vi "ovenCtrl_Na.vi"(6 "Error In (no error)":errorcluster, 9 "Temperature Log Interval (s)":dbl=20.0, 10 "Port Number Heater 1":u16=2000, 11 "IP Address Heater 1":string="192.168.12.200") -> (0 "Error Out":errorcluster, 3 "T1 (C)":dbl=214.9 format="%.2f")   [LabVIEW 2013, in "NaOvenControlV6SubVIs.lvlib"]
uses:
  VIs/NaOvenControlV6SubVIs.lvlib
panel:
  out "Oven Ramp Down Status (ON/OFF)":bool
  in  "Process":u16(ring)=1 items=["Log Temperature", "Wait - ON - Log", "OFF - Log", "OFF - Wait -ON - Log"]
  in  "Next Weekday":bool
  in  "Year":i32=2021 min=2019 step=1
  in  "Month":i32=3 min=1 max=12 step=1
  in  "Day":i32=23 min=1 max=31 step=1
  out "Oven Ramp Up Status (ON/OFF)":bool
  out "Oven Ramp ON Time":string="7:15 AM"
  out "Oven Ramp ON Date":string="Monday, March 22, 2021"
  in  "Turn ON Minute":i32=15 min=0 max=59 step=1
  in  "Turn ON Hour":i32=7 min=0 max=23 step=1
  in  "Final Hot Heater 1 Temperature (C)":dbl=215.0 min=20.0 max=260.0 step=0.1
  in  "Ramp Up Duration (min)":dbl=120.0
  in  "Set To Room Temp?":bool
  in  "Additional Temp for Heater 2":dbl=45.0
  in  "Ramp Down Duration (min)":dbl=100.0
  in  "Final Cold Heater 1 Temperature (C)":dbl=10.0 min=5.0 max=260.0 step=0.1 format="%.2f"
  out "Update to Influx (T2)":bool
  out "Update to Influx (T1)":bool
  out "T2 (C)":dbl=260.0 format="%.2f"
  in  "Port Number Heater 2":u16=2000
  in  "IP Address Heater 2":string="192.168.12.201"
  # "Common Inputs"
  # "Outputs"
  # "The Temperature and Influx update status is disabled during Ramp Up and Down"
  # "Turn ON Inputs"
  # "Ramp ON time is not visible when not scheduled"
  # "Tun OFF Inputs"
  # "Diagnosis"
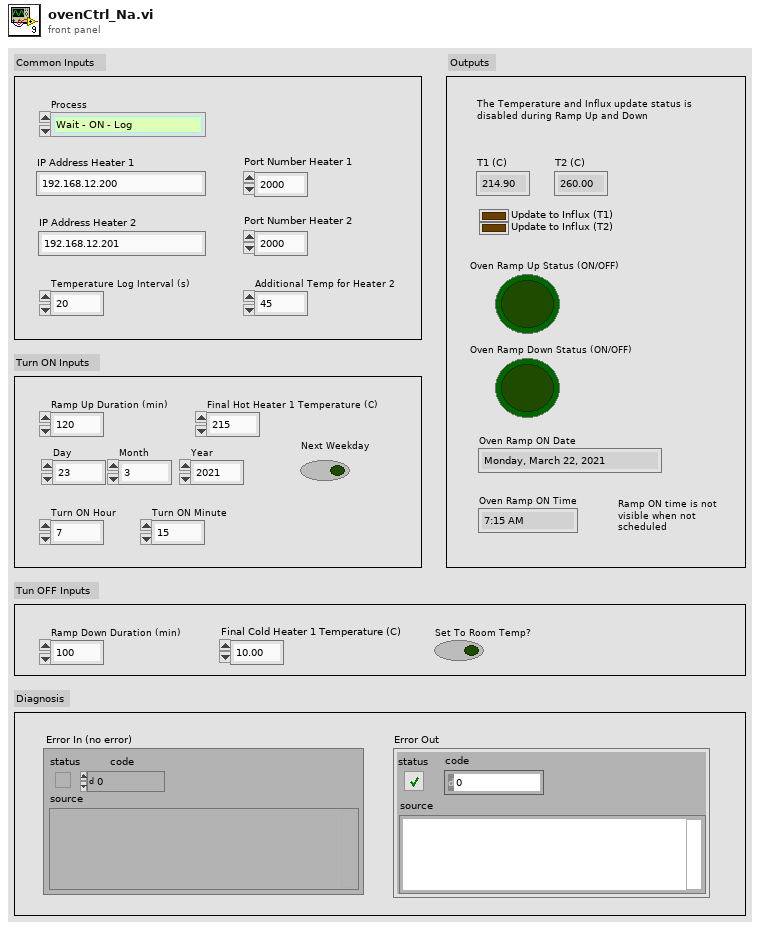
[diagram p1: front panel]
types:
  T1 = typedef "LVDateTimeRec.ctl" = cluster{"fractional second":dbl, "second":i32, "minute":i32, "hour":i32, "day of month":i32, "month":i32, "year":i32, "day of week":i32, "day of year":i32, "DST":i32}
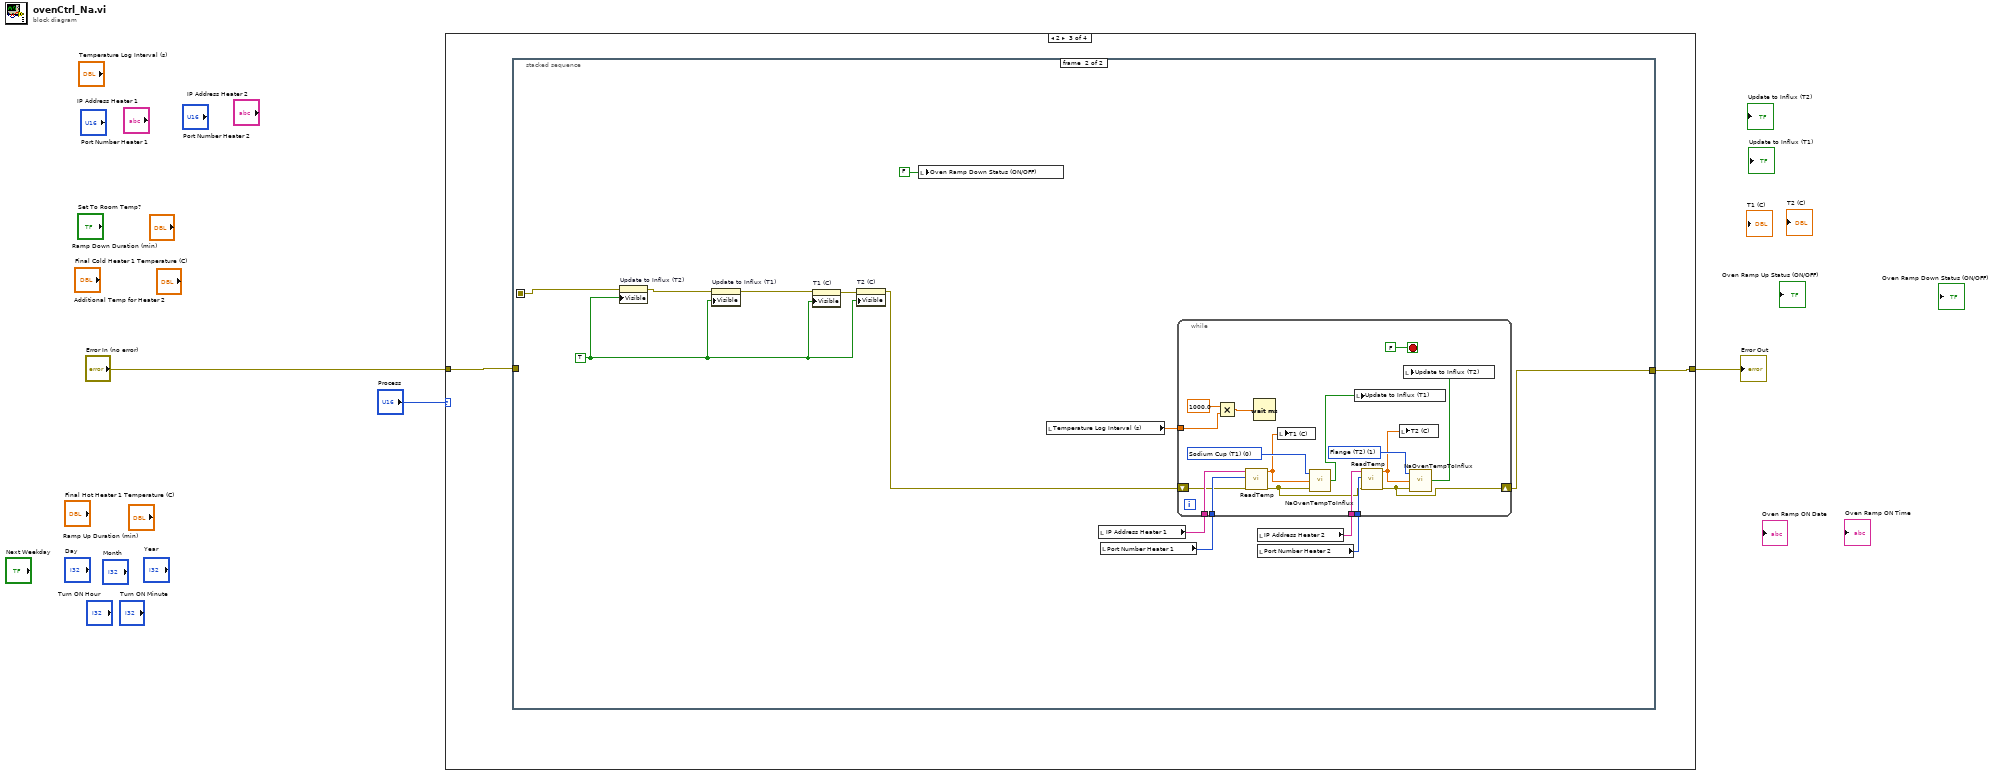
[diagram p0: block diagram]
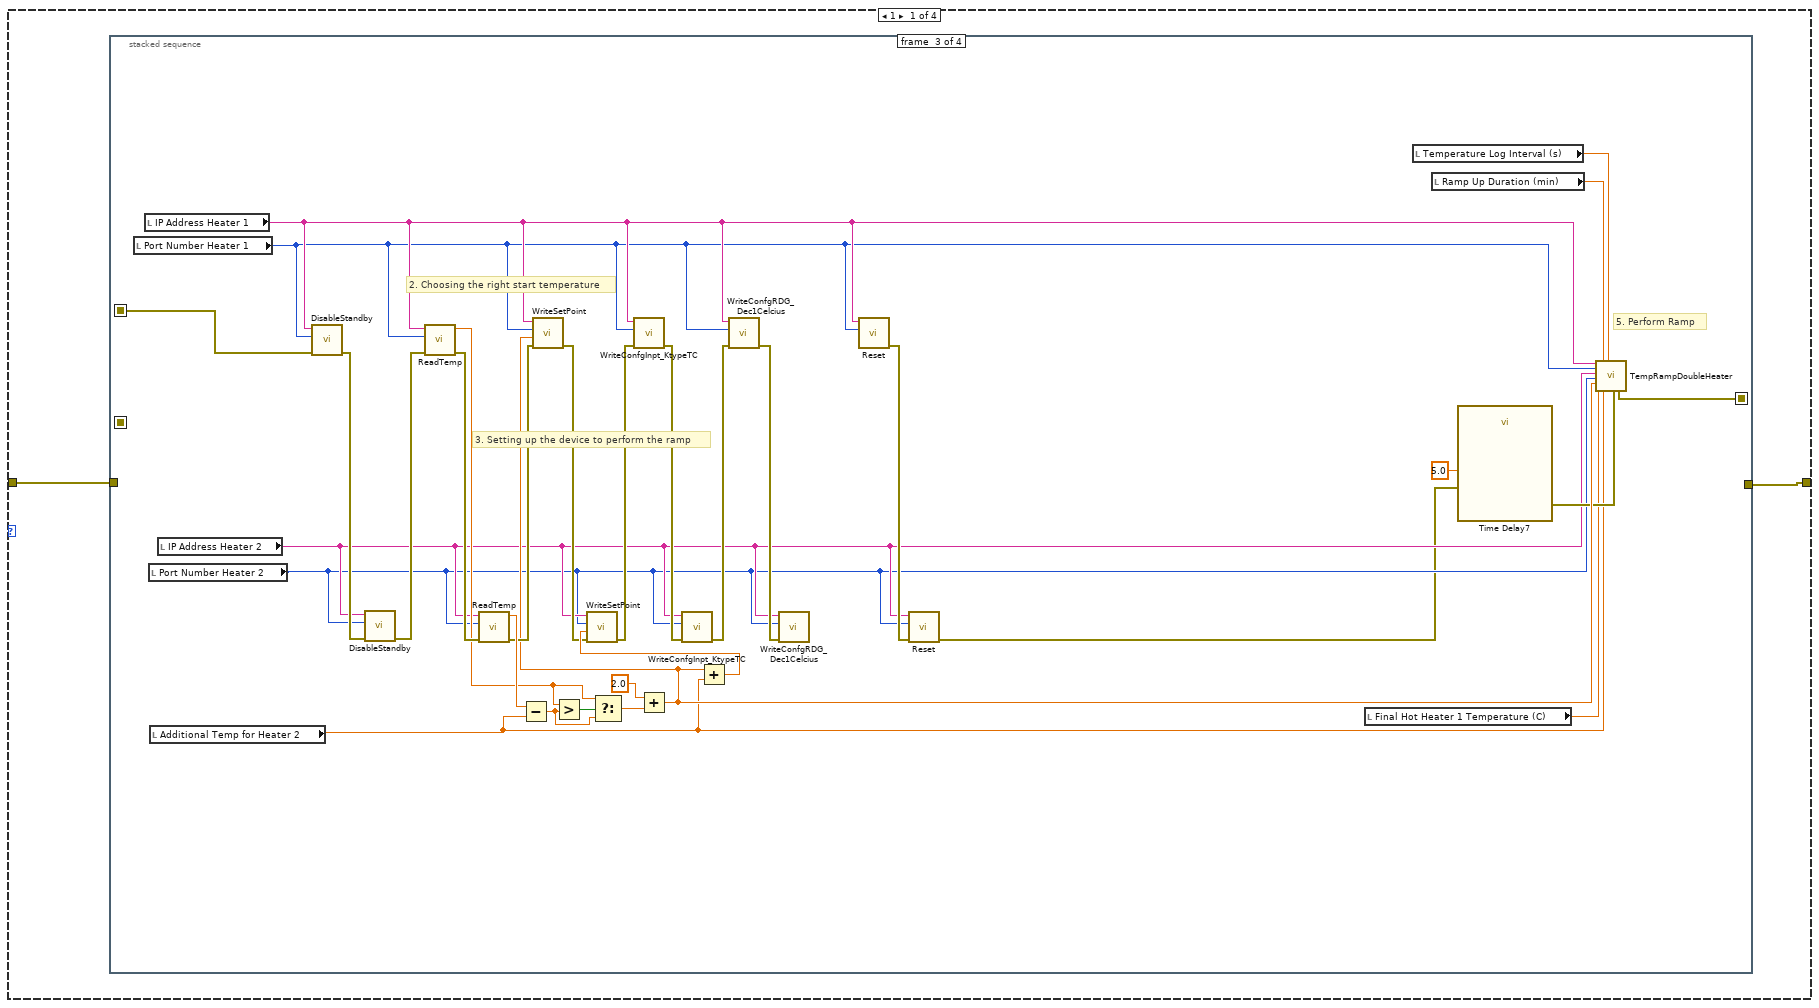
[diagram p2: hidden frame]
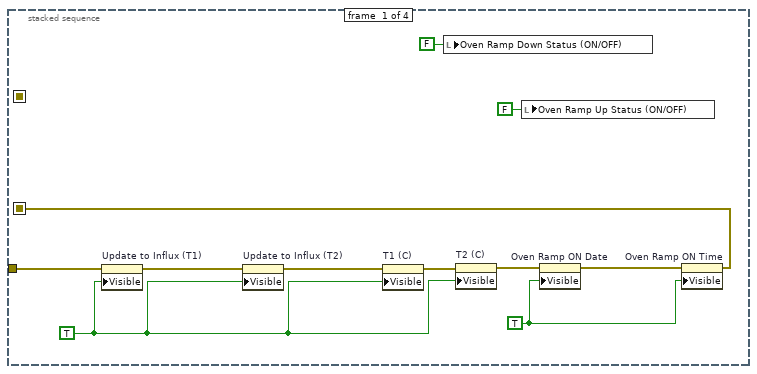
[diagram p3: hidden frame]
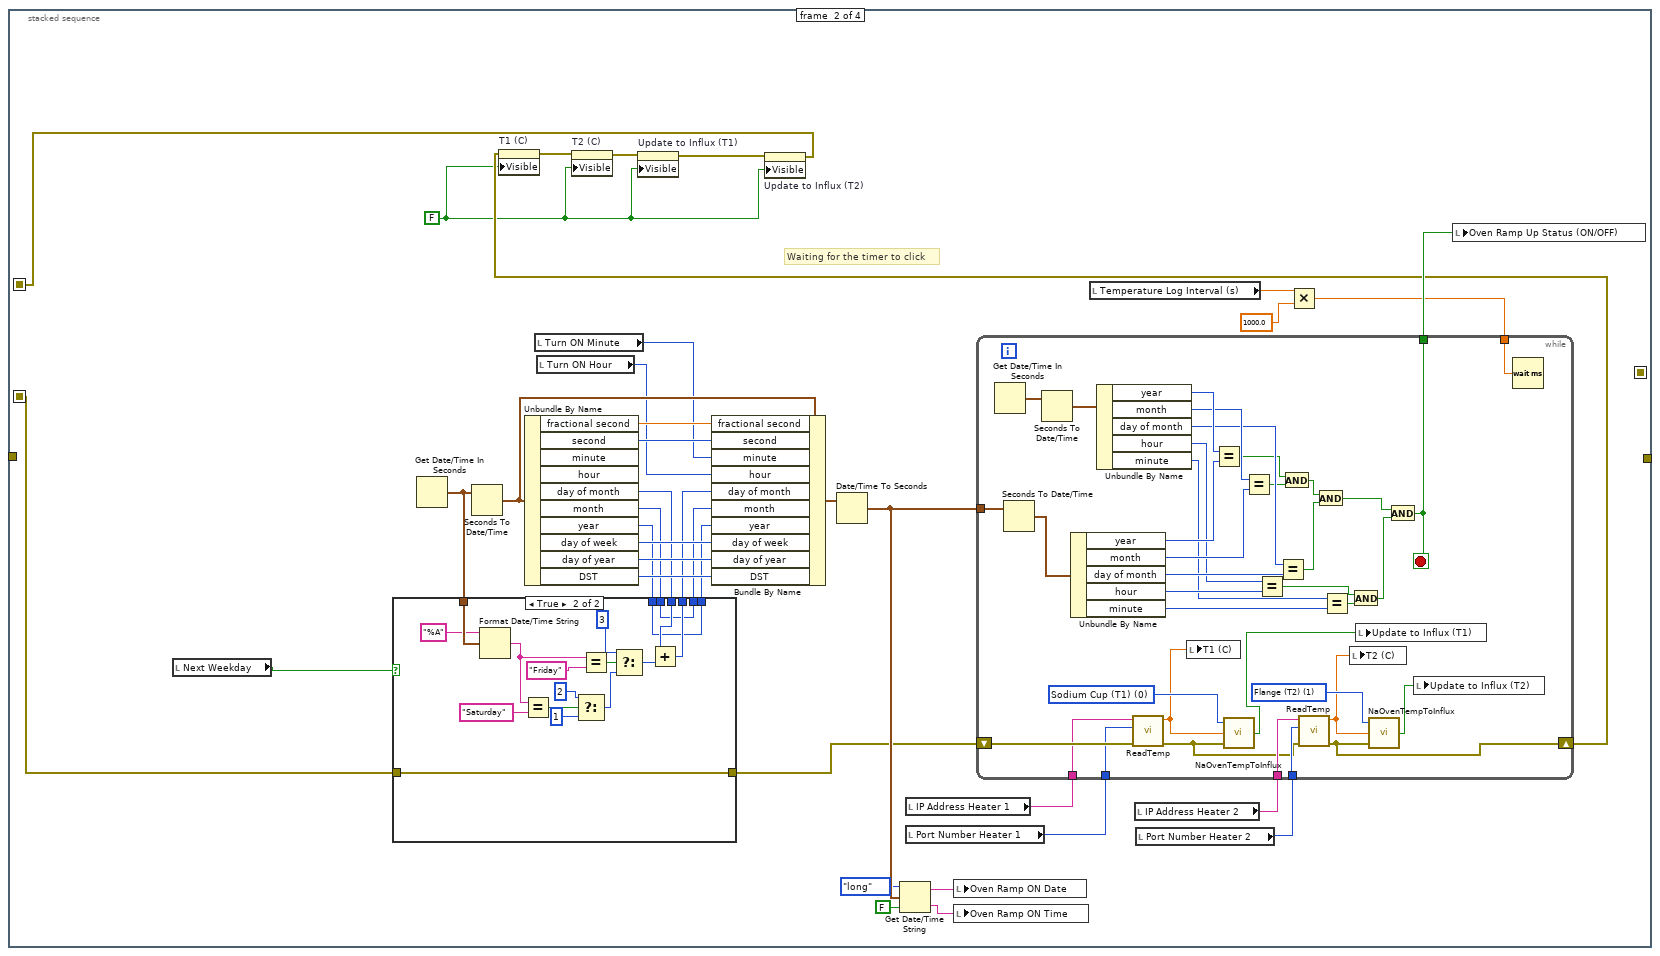
[diagram p4: hidden frame]
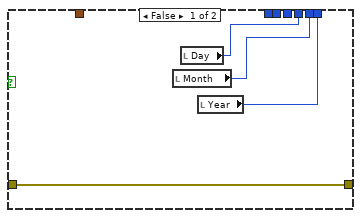
[diagram p5: hidden frame]
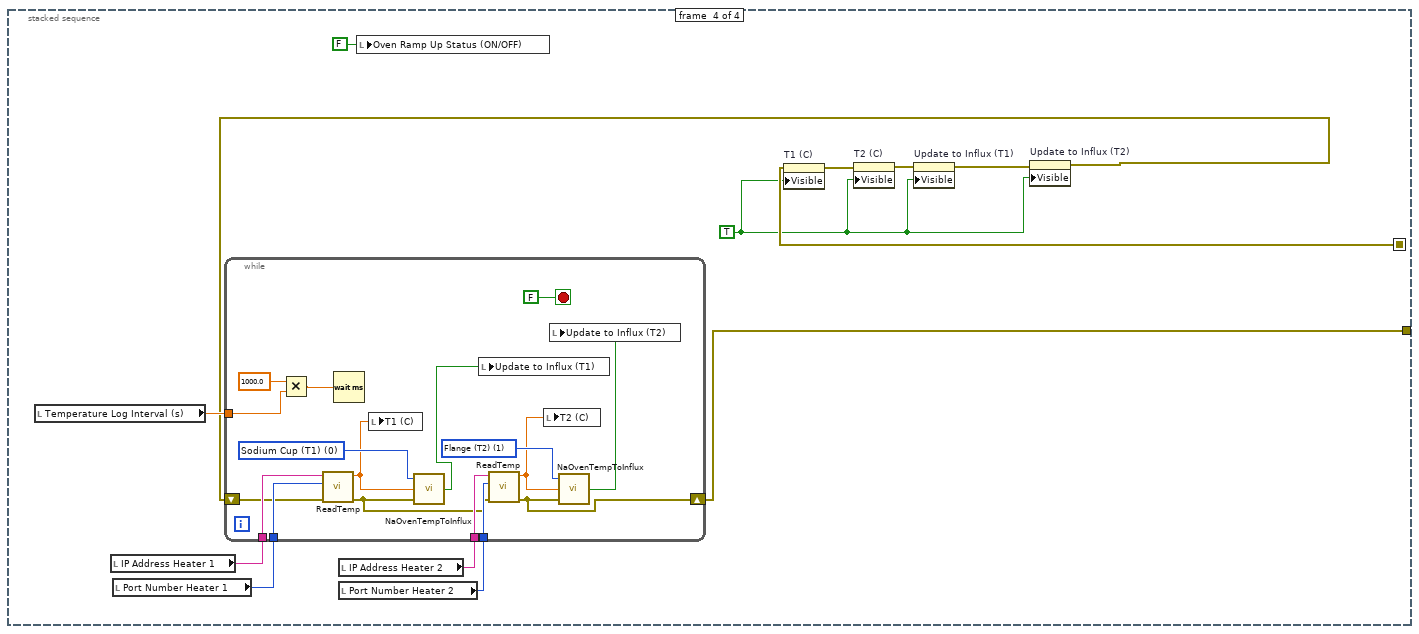
[diagram p6: hidden frame]
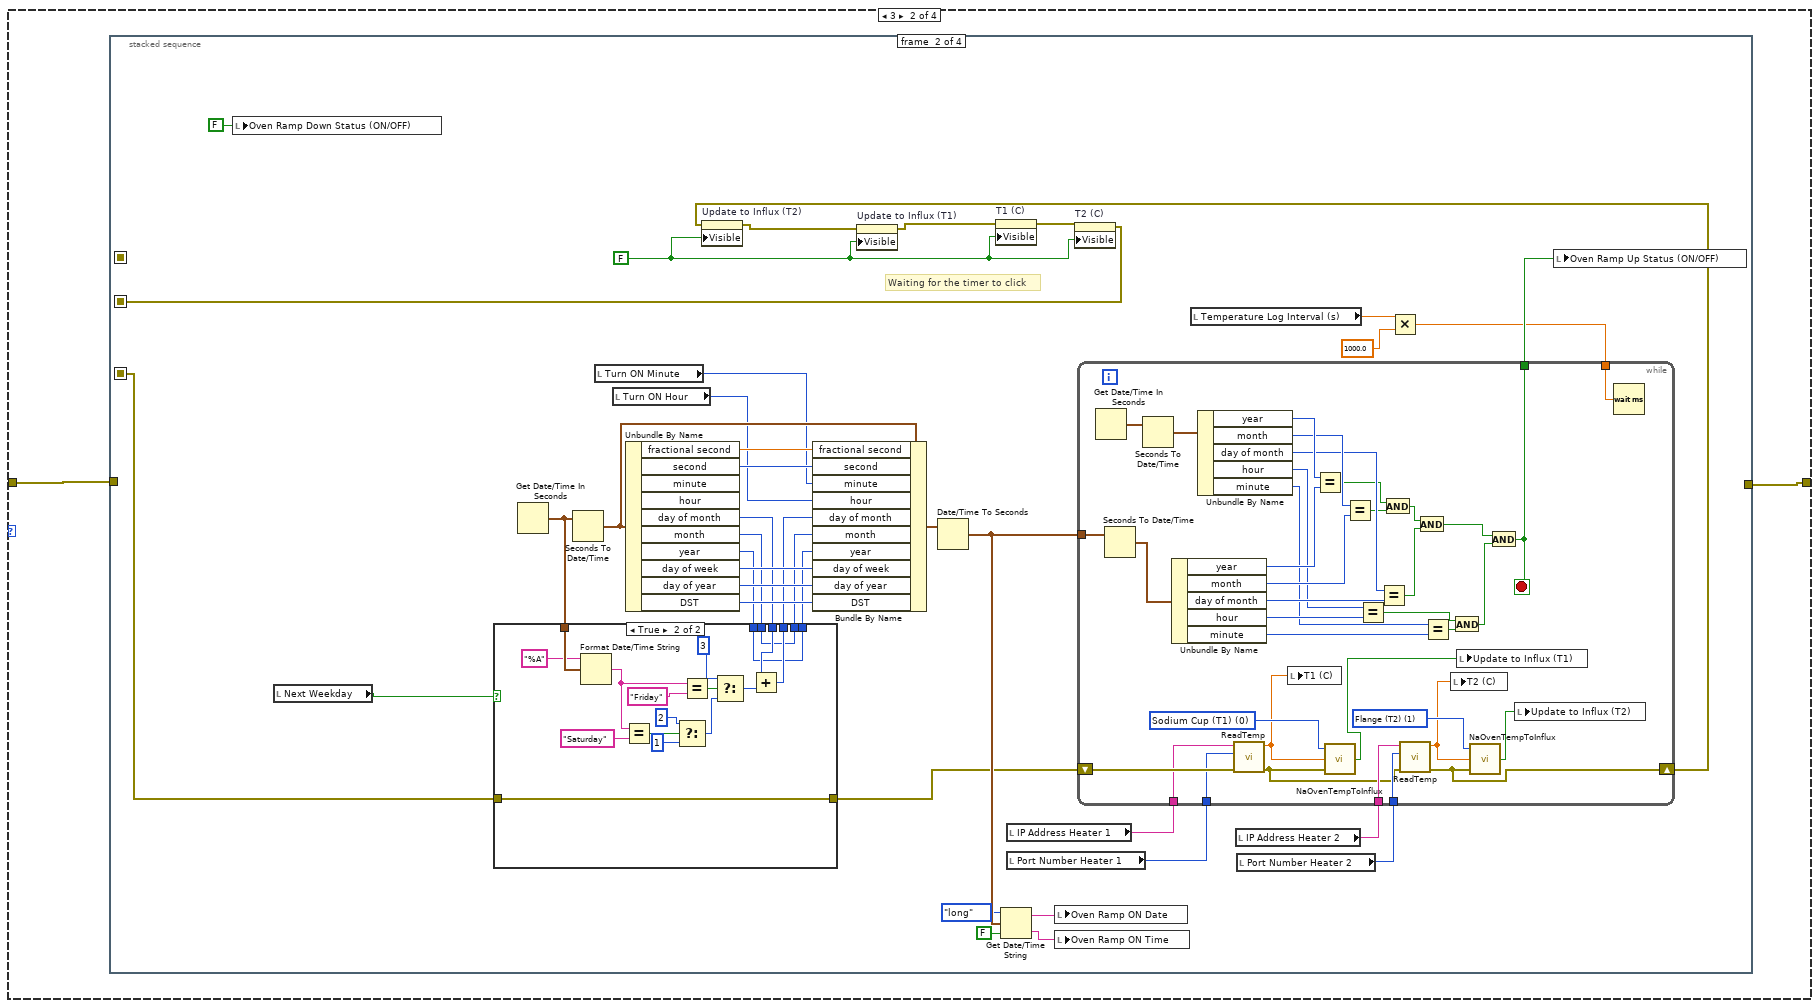
[diagram p7: hidden frame]
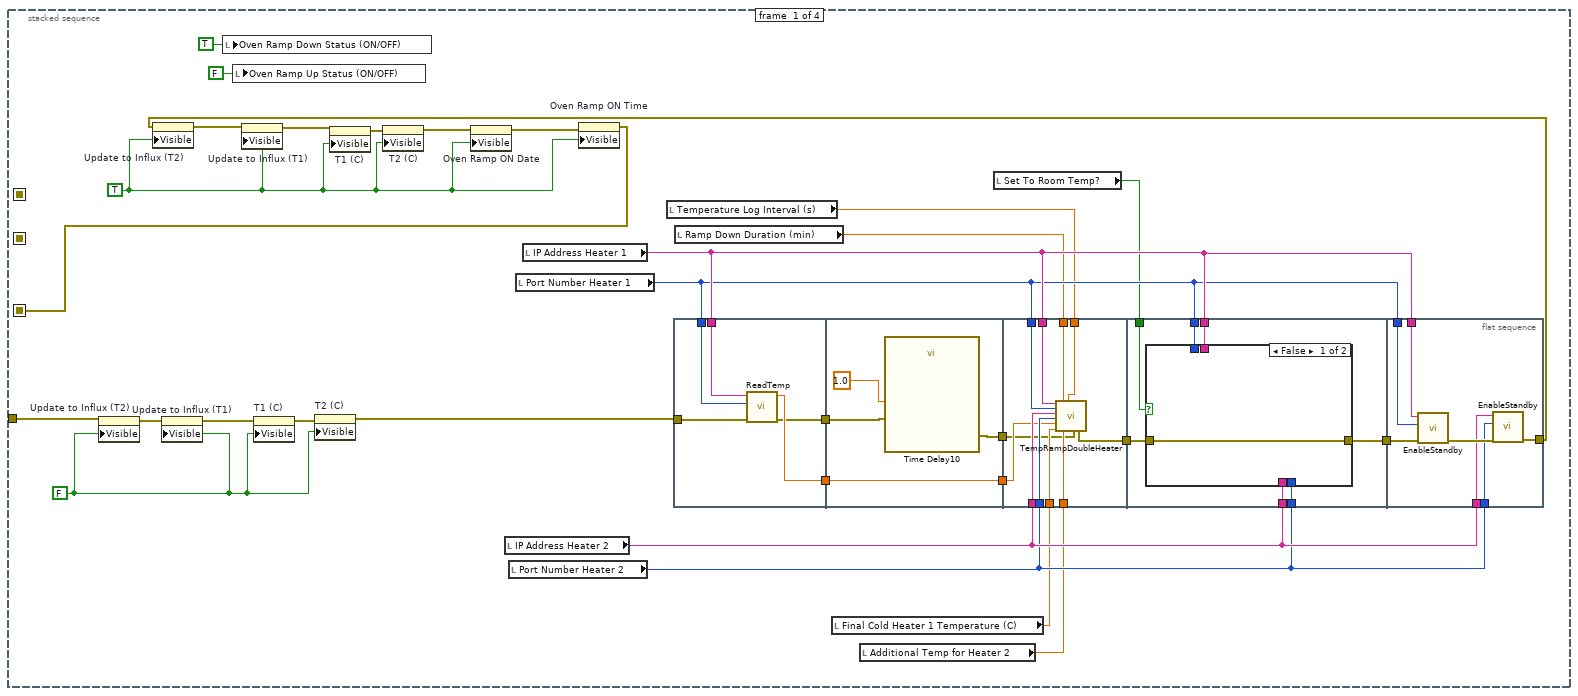
[diagram p8: hidden frame]
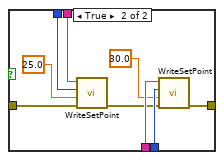
[diagram p9: hidden frame]
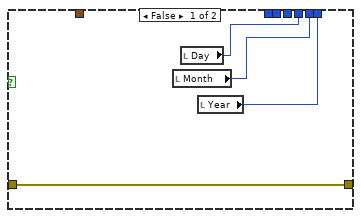
[diagram p10: hidden frame]
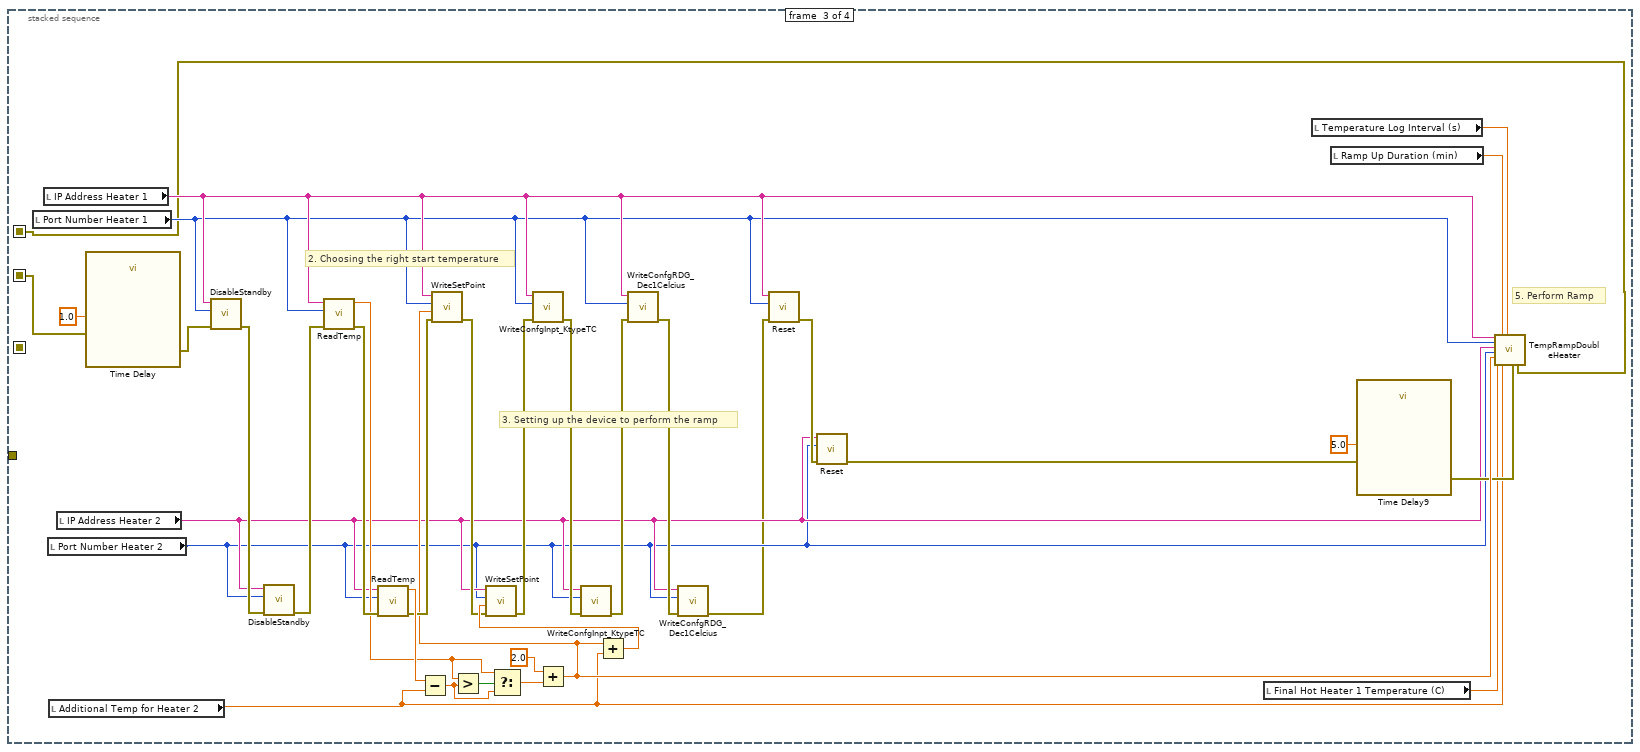
[diagram p11: hidden frame]
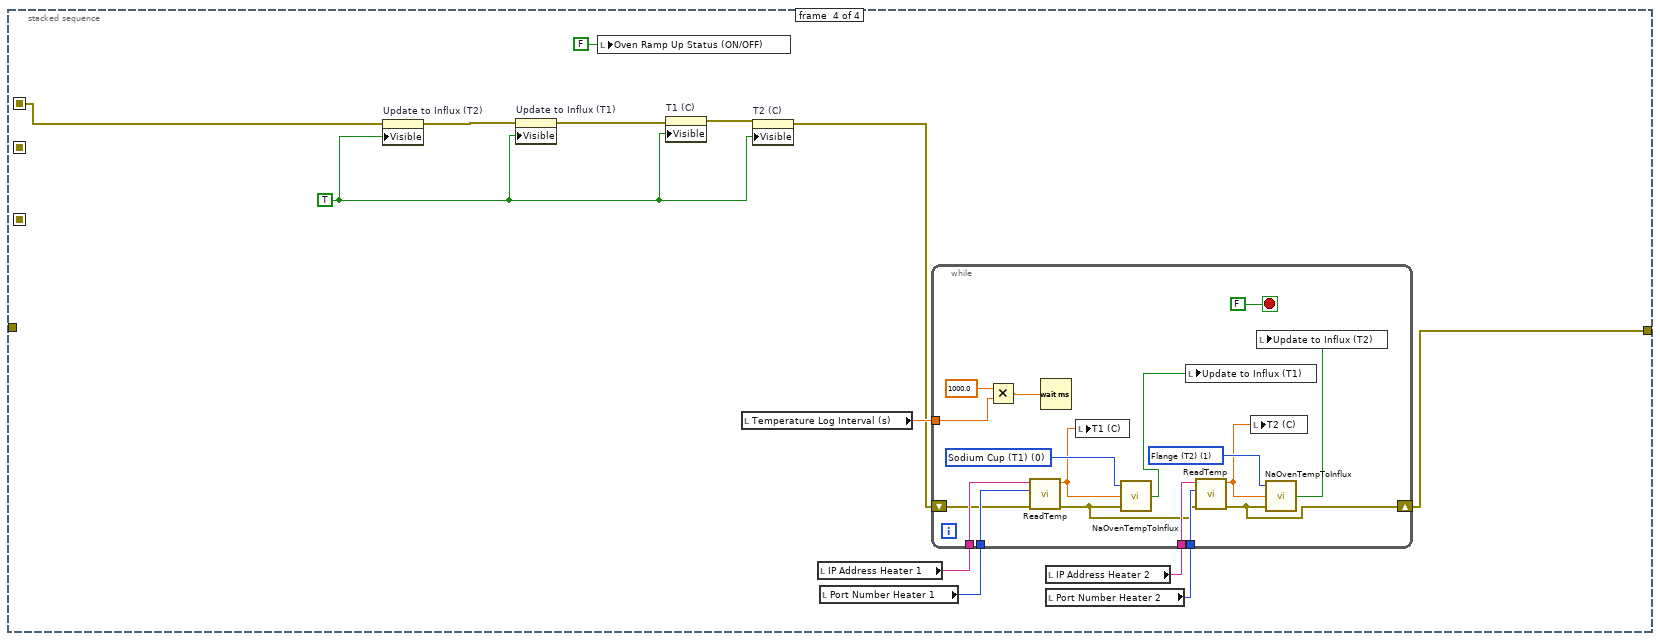
[diagram p12: hidden frame]
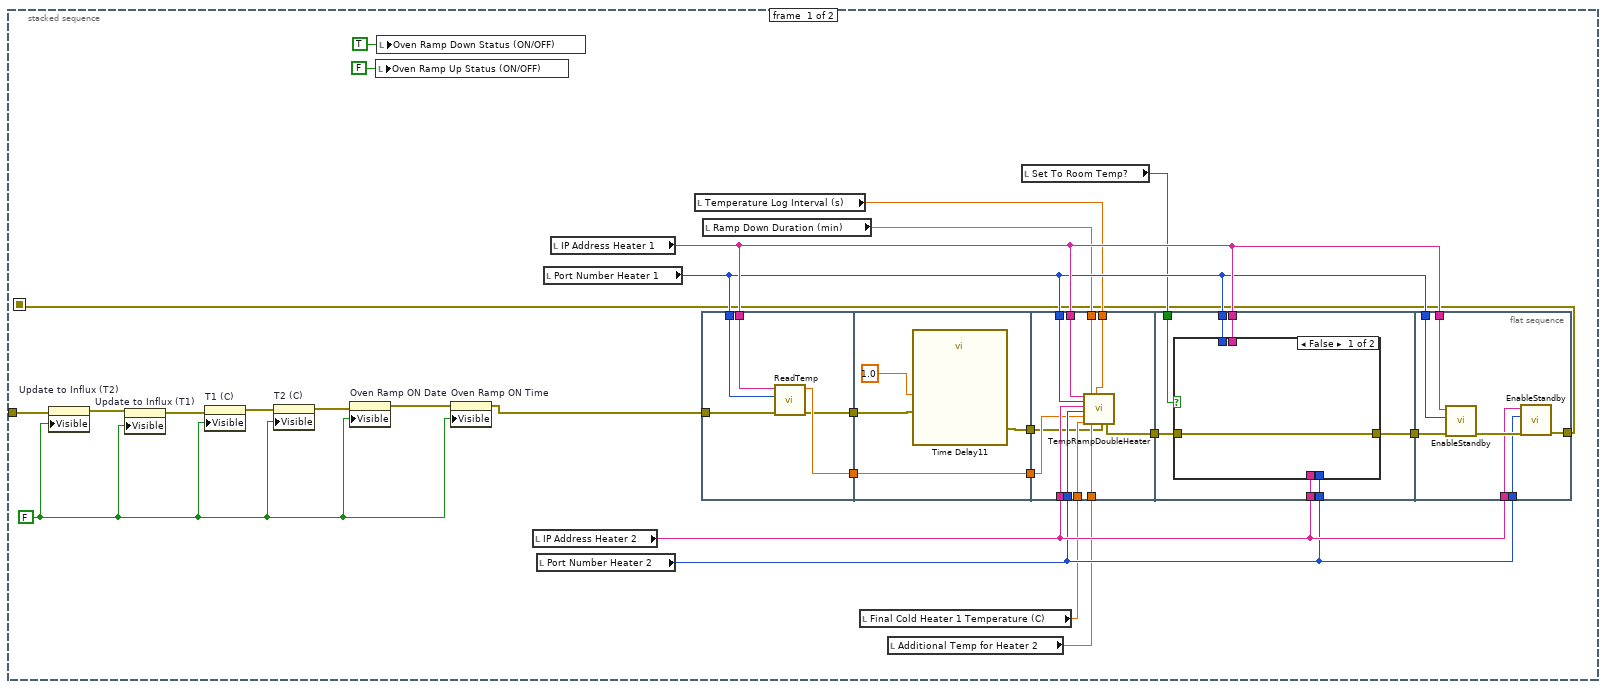
[diagram p13: hidden frame]
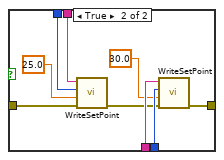
[diagram p14: hidden frame]
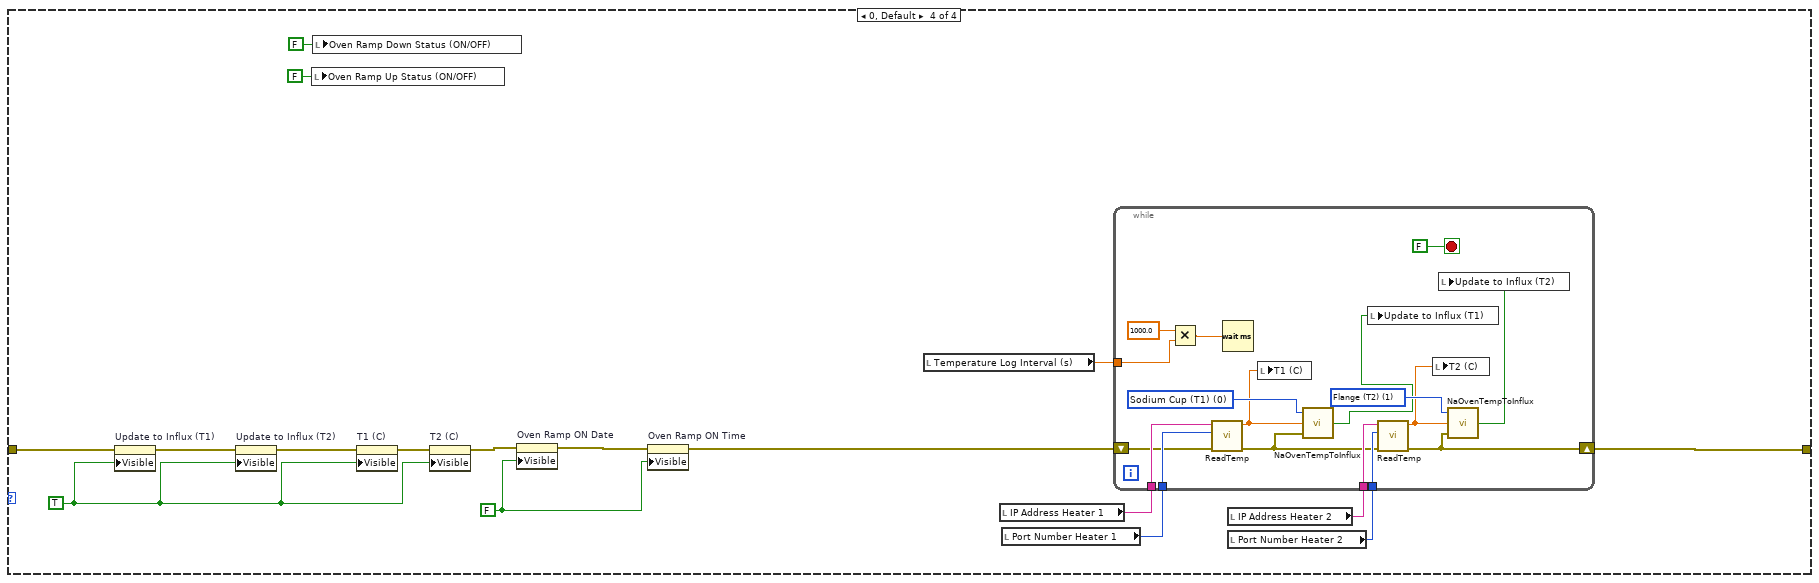
[diagram p15: hidden frame]
diagram:
  n1 = case shown="2" "Process" {
    tunnel: [w4 w174 w412 w530] -> w3
    tunnel: "Error In (no error)" -> [w5 w175 w413 w522]
    frame 1 {
      n2 = stacked-sequence {
        seq-local: [_ w18 _ _] -> [_ _ w115 _]
        seq-local: [_ _ w114 _] -> [_ _ _ w149]
        seq-local: [w7 _ _ _] -> [_ w25 _ _]
        tunnel: w5 -> [w14 _ _ _]
        tunnel: [_ _ _ w151] -> w4
        frame #0 {
          w6 = TRUE ("Visible")
          w10 = TRUE ("Visible")
          n3 = property on="Update to Influx (T1)" class="Bool (strict)"(error in=w14, "Visible"=w10) -> (error out=w13:errorcluster)  [unwired: 1 in, 1 out]
          n4 = property on="Update to Influx (T2)" class="Bool (strict)"(error in=w13, "Visible"=w10) -> (error out=w12:errorcluster)  [unwired: 1 in, 1 out]
          n5 = property on="T1 (C)" class="DigNum (strict)"(error in=w12, "Visible"=w10) -> (error out=w11:errorcluster)  [unwired: 1 in, 1 out]
          n6 = local write "Oven Ramp Down Status (ON/OFF)"(FALSE ("Oven Ramp Down Status (ON/OFF)")) -> ()
          n7 = property on="T2 (C)" class="DigNum (strict)"(error in=w11, "Visible"=w10) -> (error out=w9:errorcluster)  [unwired: 1 in, 1 out]
          n8 = local write "Oven Ramp Up Status (ON/OFF)"(FALSE ("Oven Ramp Up Status (ON/OFF)")) -> ()
          n9 = property on="Oven Ramp ON Date" class="Str"(error in=w9, "Visible"=w6) -> (error out=w8:errorcluster)  [unwired: 1 in, 1 out]
          n10 = property on="Oven Ramp ON Time" class="Str"(error in=w8, "Visible"=w6) -> (error out=w7:errorcluster)  [unwired: 1 in, 1 out]
        }
        frame #1 {
          w17 = FALSE ("Visible")
          # "Waiting for the timer to click"
          n11 = local read "Next Weekday"() -> (w35:bool)
          n12 = Get Date/Time In Seconds() -> (seconds since 1Jan1904=w47:timestamp)
          n13 = Seconds To Date/Time(time stamp (now)=w47) -> (date time rec=w49:T1)  [unwired: 1 in]
          n14 = Unbundle By Name(w49) -> ("fractional second"=w54:dbl, "second"=w53:i32, "day of month"=w46:i32, "month"=w44:i32, "year"=w42:i32, "day of week"=w52:i32, "day of year"=w51:i32, "DST"=w50:i32)  [unwired: 2 out]
          n15 = case shown="True" w35 {
            tunnel: w47 -> [_ w75]
            tunnel: w46 -> [_ w64]
            tunnel: [w57 w62] -> w45
            tunnel: w44 -> [_ w61]
            tunnel: [w56 w61] -> w43
            tunnel: w42 -> [_ w60]
            tunnel: [w55 w60] -> w41
            tunnel: w25 -> [w58 w59]
            tunnel: [w58 w59] -> w36
            frame False {
              n16 = local read "Month"() -> (w56:i32)
              n17 = local read "Day"() -> (w57:i32)
              n18 = local read "Year"() -> (w55:i32)
            }
            frame True {
              n19 = Format Date/Time String(time format string (%c)="%A", seconds (now)=w75) -> (date/time string=w72:string)  [unwired: 1 in]
              n20 = Equal?(x=w72, y="Saturday") -> (x = y?=w68:bool)
              n21 = Select(t=2, s=w68, f=1) -> (s? t:f=w65:i32)
              n22 = Equal?(x=w72, y="Friday") -> (x = y?=w70:bool)
              n23 = Select(t=3, s=w70, f=w65) -> (s? t:f=w63:i32)
              n24 = Add(x=w64, y=w63) -> (x+y=w62:i32)
            }
          }
          n25 = local read "Turn ON Minute"() -> (w24:i32)
          n26 = local read "Turn ON Hour"() -> (w23:i32)
          n27 = Bundle By Name(cluster=w49, "fractional second"=w54, "second"=w53, "minute"=w24, "hour"=w23, "day of month"=w45, "month"=w43, "year"=w41, "day of week"=w52, "day of year"=w51, "DST"=w50) -> (w48:T1)
          n28 = Date/Time To Seconds(2:w48) -> (0:w39:timestamp)  [unwired: 1 in]
          n29 = Get Date/Time String(date format (0)=enum16{"short", "long", "abbreviated"}."long", seconds (now)=w39, want seconds? (F)=FALSE) -> (date string=w34:string, time string=w33:string)
          n30 = local read "IP Address Heater 1"() -> (w29:string)
          n31 = local read "Port Number Heater 1"() -> (w28:u16)
          n32 = local write "Oven Ramp ON Date"(w34) -> ()
          n33 = local write "Oven Ramp ON Time"(w33) -> ()
          n34 = local read "Temperature Log Interval (s)"() -> (w31:dbl)
          n35 = local read "IP Address Heater 2"() -> (w26:string)
          n36 = local read "Port Number Heater 2"() -> (w27:u16)
          n37 = Multiply(x=w31, y=1000.0) -> (x*y=w30:dbl)
          n38 = while {
            tunnel: w39 -> [w111]
            tunnel: [w90] -> w40
            shift-right: [w76] -> w22
            shift-left: w36 -> [w86]
            tunnel: w30 -> [w89]
            tunnel: w29 -> [w83]
            tunnel: w28 -> [w82]
            tunnel: w27 -> [w81]
            tunnel: w26 -> [w80]
            stop <- w90 stop-if-true
            w87 = u16 1 items=["Sodium Cup (T1)", "Flange (T2)"] ("Thermocouple")
            w88 = u16 0 items=["Sodium Cup (T1)", "Flange (T2)"] ("Thermocouple")
            n39 = Get Date/Time In Seconds() -> (seconds since 1Jan1904=w112:timestamp)
            n40 = Seconds To Date/Time(time stamp (now)=w111) -> (date time rec=w110:T1)  [unwired: 1 in]
            n41 = Seconds To Date/Time(time stamp (now)=w112) -> (date time rec=w109:T1)  [unwired: 1 in]
            n42 = Unbundle By Name(w110) -> ("year"=w107:i32, "month"=w105:i32, "day of month"=w103:i32, "hour"=w101:i32, "minute"=w99:i32)
            n43 = Unbundle By Name(w109) -> ("year"=w108:i32, "month"=w106:i32, "day of month"=w104:i32, "hour"=w102:i32, "minute"=w100:i32)
            n44 = call "ReadTemp.vi"("error in (no error)"=w86, "Port Number"=w82, "IP Address"=w83) -> ("error out"=w77:errorcluster, "Temperature"=w85:dbl)  [unwired: 7 in]
            n45 = local write "T1 (C)"(w85) -> ()
            n46 = Equal?(x=w108, y=w107) -> (x = y?=w98:bool)
            n47 = call "NaOvenTempToInflux.vi"("error in (no error)"=w77, "Temperature Input"=w85, "Thermocouple"=w88) -> ("InfluxDB Comm Error"=w79:bool)  [unwired: 1 in, 1 out]
            n48 = Equal?(x=w106, y=w105) -> (x = y?=w97:bool)
            n49 = Equal?(x=w102, y=w101) -> (x = y?=w96:bool)
            n50 = Equal?(x=w104, y=w103) -> (x = y?=w93:bool)
            n51 = And(x=w98, y=w97) -> (x .and. y?=w94:bool)
            n52 = call "ReadTemp.vi"("error in (no error)"=w77, "Port Number"=w81, "IP Address"=w80) -> ("error out"=w76:errorcluster, "Temperature"=w84:dbl)  [unwired: 7 in]
            n53 = And(x=w94, y=w93) -> (x .and. y?=w92:bool)
            n54 = Equal?(x=w100, y=w99) -> (x = y?=w95:bool)
            n55 = local write "T2 (C)"(w84) -> ()
            n56 = And(x=w96, y=w95) -> (x .and. y?=w91:bool)
            n57 = local write "Update to Influx (T1)"(w79) -> ()
            n58 = call "NaOvenTempToInflux.vi"("error in (no error)"=w76, "Temperature Input"=w84, "Thermocouple"=w87) -> ("InfluxDB Comm Error"=w78:bool)  [unwired: 1 in, 1 out]
            n59 = And(x=w92, y=w91) -> (x .and. y?=w90:bool)
            n60 = local write "Update to Influx (T2)"(w78) -> ()
            n61 = Wait (ms)(milliseconds to wait=w89) -> ()  [unwired: 1 out]
          }
          n62 = property on="T1 (C)" class="DigNum (strict)"(error in=w22, "Visible"=w17) -> (error out=w21:errorcluster)  [unwired: 1 in, 1 out]
          n63 = property on="T2 (C)" class="DigNum (strict)"(error in=w21, "Visible"=w17) -> (error out=w20:errorcluster)  [unwired: 1 in, 1 out]
          n64 = property on="Update to Influx (T1)" class="Bool (strict)"(error in=w20, "Visible"=w17) -> (error out=w19:errorcluster)  [unwired: 1 in, 1 out]
          n65 = property on="Update to Influx (T2)" class="Bool (strict)"(error in=w19, "Visible"=w17) -> (error out=w18:errorcluster)  [unwired: 1 in, 1 out]
          n66 = local write "Oven Ramp Up Status (ON/OFF)"(w40) -> ()
        }
        frame #2 {
          # "5. Perform Ramp"
          # "3. Setting up the device to perform the ramp"
          # "2. Choosing the right start temperature"
          n67 = local read "Port Number Heater 1"() -> (w122:u16)
          n68 = local read "IP Address Heater 1"() -> (w123:string)
          n69 = local read "Port Number Heater 2"() -> (w120:u16)
          n70 = local read "Additional Temp for Heater 2"() -> (w119:dbl)
          n71 = local read "IP Address Heater 2"() -> (w121:string)
          n72 = call "DisableStandby.vi"("error in (no error)"=w115, "Port Number"=w122, "IP Address"=w123) -> ("error out"=w125:errorcluster)  [unwired: 7 in, 1 out]
          n73 = call "DisableStandby.vi"("error in (no error)"=w125, "Port Number"=w120, "IP Address"=w121) -> ("error out"=w124:errorcluster)  [unwired: 7 in, 1 out]
          n74 = call "ReadTemp.vi"("error in (no error)"=w124, "Port Number"=w122, "IP Address"=w123) -> ("error out"=w136:errorcluster, "Temperature"=w133:dbl)  [unwired: 7 in]
          n75 = call "ReadTemp.vi"("error in (no error)"=w136, "Port Number"=w120, "IP Address"=w121) -> ("error out"=w131:errorcluster, "Temperature"=w135:dbl)  [unwired: 7 in]
          n76 = Subtract(x=w135, y=w119) -> (x-y=w132:dbl)
          n77 = Greater?(x=w133, y=w132) -> (0:w134:bool)
          n78 = Select(t=w133, s=w134, f=w132) -> (s? t:f=w130:dbl)
          n79 = Add(x=2.0, y=w130) -> (x+y=w128:dbl)
          n80 = call "WriteSetPoint.vi"("error in (no error)"=w131, "Setpoint (C)"=w128, "Port Number"=w122, "IP Address"=w123) -> ("error out"=w142:errorcluster)  [unwired: 6 in, 1 out]
          n81 = Add(x=w128, y=w119) -> (x+y=w143:dbl)
          n82 = call "WriteSetPoint.vi"("error in (no error)"=w142, "Setpoint (C)"=w143, "Port Number"=w120, "IP Address"=w121) -> ("error out"=w141:errorcluster)  [unwired: 6 in, 1 out]
          n83 = call "WriteConfgInpt_KtypeTC.vi"("error in (no error)"=w141, "Port Number"=w122, "IP Address"=w123) -> ("error out"=w140:errorcluster)  [unwired: 7 in, 1 out]
          n84 = call "WriteConfgInpt_KtypeTC.vi"("error in (no error)"=w140, "Port Number"=w120, "IP Address"=w121) -> ("error out"=w139:errorcluster)  [unwired: 7 in, 1 out]
          n85 = call "WriteConfgRDG_Dec1Celcius.vi"("error in (no error)"=w139, "Port Number"=w122, "IP Address"=w123) -> ("error out"=w138:errorcluster)  [unwired: 7 in, 1 out]
          n86 = call "WriteConfgRDG_Dec1Celcius.vi"("error in (no error)"=w138, "Port Number"=w120, "IP Address"=w121) -> ()  [unwired: 7 in, 2 out]
          n87 = call "Reset.vi"("Port Number"=w122, "IP Address"=w123) -> ("error out"=w137:errorcluster)  [unwired: 8 in, 1 out]
          n88 = call "Reset.vi"("error in (no error)"=w137, "Port Number"=w120, "IP Address"=w121) -> ("error out"=w113:errorcluster)  [unwired: 7 in, 1 out]
          n89 = local read "Final Hot Heater 1 Temperature (C)"() -> (w116:dbl)
          n90 = local read "Temperature Log Interval (s)"() -> (w117:dbl)
          n91 = local read "Ramp Up Duration (min)"() -> (w118:dbl)
          n92 = call "Time Delay7"("error in (no error)"=w113, "Delay Time (s)"=5.0) -> ("error out"=w127:errorcluster)  [unwired: 9 in]
          n93 = call "TempRampDoubleHeater.vi"("IP Address Heater 1"=w123, "Port Number Heater 1"=w122, "IP Address Heater 2"=w121, "Port Number Heater 2"=w120, "Start T1 (C)"=w128, "End T1 (C)"=w116, "Duration of Ramp (min)"=w118, "Additional Temperature for Heater 2"=w119, "Temperature Log Interval (s)"=w117, "Error In (no error)"=w127) -> ("Error Out"=w114:errorcluster)  [unwired: 3 in, 6 out]
        }
        frame #3 {
          w145 = TRUE ("Visible")
          n94 = local read "Temperature Log Interval (s)"() -> (w156:dbl)
          n95 = local read "IP Address Heater 1"() -> (w155:string)
          n96 = local read "Port Number Heater 1"() -> (w154:u16)
          n97 = local read "IP Address Heater 2"() -> (w153:string)
          n98 = local read "Port Number Heater 2"() -> (w152:u16)
          n99 = local write "Oven Ramp Up Status (ON/OFF)"(FALSE ("Oven Ramp Up Status (ON/OFF)")) -> ()
          n100 = property on="T1 (C)" class="DigNum (strict)"(error in=w149, "Visible"=w145) -> (error out=w148:errorcluster)  [unwired: 1 in, 1 out]
          n101 = property on="T2 (C)" class="DigNum (strict)"(error in=w148, "Visible"=w145) -> (error out=w147:errorcluster)  [unwired: 1 in, 1 out]
          n102 = property on="Update to Influx (T1)" class="Bool (strict)"(error in=w147, "Visible"=w145) -> (error out=w146:errorcluster)  [unwired: 1 in, 1 out]
          n103 = property on="Update to Influx (T2)" class="Bool (strict)"(error in=w146, "Visible"=w145) -> (error out=w144:errorcluster)  [unwired: 1 in, 1 out]
          n104 = while {
            tunnel: w156 -> [w170]
            tunnel: w155 -> [w172]
            tunnel: w154 -> [w171]
            shift-right: [w157] -> w151
            shift-left: w144 -> [w168]
            tunnel: w153 -> [w166]
            tunnel: w152 -> [w165]
            stop <- FALSE stop-if-true
            w163 = u16 1 items=["Sodium Cup (T1)", "Flange (T2)"] ("Thermocouple")
            w164 = u16 0 items=["Sodium Cup (T1)", "Flange (T2)"] ("Thermocouple")
            n105 = Multiply(x=1000.0 ("y"), y=w170) -> (x*y=w173:dbl)
            n106 = call "ReadTemp.vi"("error in (no error)"=w168, "Port Number"=w171, "IP Address"=w172) -> ("error out"=w158:errorcluster, "Temperature"=w162:dbl)  [unwired: 7 in]
            n107 = Wait (ms)(milliseconds to wait=w173) -> ()  [unwired: 1 out]
            n108 = local write "T1 (C)"(w162) -> ()
            n109 = call "NaOvenTempToInflux.vi"("error in (no error)"=w158, "Temperature Input"=w162, "Thermocouple"=w164) -> ("InfluxDB Comm Error"=w160:bool)  [unwired: 1 in, 1 out]
            n110 = local write "Update to Influx (T1)"(w160) -> ()
            n111 = call "ReadTemp.vi"("error in (no error)"=w158, "Port Number"=w165, "IP Address"=w166) -> ("error out"=w157:errorcluster, "Temperature"=w161:dbl)  [unwired: 7 in]
            n112 = local write "T2 (C)"(w161) -> ()
            n113 = call "NaOvenTempToInflux.vi"("error in (no error)"=w157, "Temperature Input"=w161, "Thermocouple"=w163) -> ("InfluxDB Comm Error"=w159:bool)  [unwired: 1 in, 1 out]
            n114 = local write "Update to Influx (T2)"(w159) -> ()
          }
        }
      }
    }
    frame 3 {
      n115 = stacked-sequence {
        seq-local: [w177 _ _ _] -> [_ w258 _ _]
        seq-local: [_ w256 _ _] -> [_ _ w350 _]
        seq-local: [_ _ w352 _] -> [_ _ _ w387]
        tunnel: w175 -> [w189 _ _ _]
        tunnel: [_ _ _ w389] -> w174
        frame #0 {
          w176 = TRUE ("Visible")
          w185 = FALSE ("Visible")
          n116 = property on="Update to Influx (T2)" class="Bool (strict)"(error in=w189, "Visible"=w185) -> (error out=w188:errorcluster)  [unwired: 1 in, 1 out]
          n117 = property on="Update to Influx (T2)" class="Bool (strict)"(error in=w184, "Visible"=w176) -> (error out=w183:errorcluster)  [unwired: 1 in, 1 out]
          n118 = property on="Update to Influx (T1)" class="Bool (strict)"(error in=w188, "Visible"=w185) -> (error out=w187:errorcluster)  [unwired: 1 in, 1 out]
          n119 = local write "Oven Ramp Down Status (ON/OFF)"(TRUE ("Oven Ramp Down Status (ON/OFF)")) -> ()
          n120 = local write "Oven Ramp Up Status (ON/OFF)"(FALSE ("Oven Ramp Up Status (ON/OFF)")) -> ()
          n121 = property on="Update to Influx (T1)" class="Bool (strict)"(error in=w183, "Visible"=w176) -> (error out=w182:errorcluster)  [unwired: 1 in, 1 out]
          n122 = property on="T1 (C)" class="DigNum (strict)"(error in=w187, "Visible"=w185) -> (error out=w186:errorcluster)  [unwired: 1 in, 1 out]
          n123 = property on="T2 (C)" class="DigNum (strict)"(error in=w186, "Visible"=w185) -> (error out=w179:errorcluster)  [unwired: 1 in, 1 out]
          n124 = property on="T1 (C)" class="DigNum (strict)"(error in=w182, "Visible"=w176) -> (error out=w181:errorcluster)  [unwired: 1 in, 1 out]
          n125 = property on="T2 (C)" class="DigNum (strict)"(error in=w181, "Visible"=w176) -> (error out=w178:errorcluster)  [unwired: 1 in, 1 out]
          n126 = property on="Oven Ramp ON Date" class="Str"(error in=w178, "Visible"=w176) -> (error out=w180:errorcluster)  [unwired: 1 in, 1 out]
          n127 = local read "IP Address Heater 2"() -> (w198:string)
          n128 = local read "Port Number Heater 2"() -> (w197:u16)
          n129 = local read "Port Number Heater 1"() -> (w199:u16)
          n130 = local read "IP Address Heater 1"() -> (w200:string)
          n131 = property on="Oven Ramp ON Time" class="Str"(error in=w180, "Visible"=w176) -> (error out=w177:errorcluster)  [unwired: 1 in, 1 out]
          n132 = local read "Temperature Log Interval (s)"() -> (w193:dbl)
          n133 = flat-sequence {
            tunnel: w200 -> [w211]
            tunnel: w199 -> [w210]
            tunnel: w179 -> [w207]
            tunnel: [w209] -> w206
            tunnel: [w208] -> w205
            tunnel: w206 -> [w215]
            tunnel: w205 -> [w213]
            tunnel: [w215] -> w204
            tunnel: [w212] -> w203
            tunnel: w204 -> [w222]
            tunnel: w200 -> [w226]
            tunnel: w199 -> [w225]
            tunnel: w198 -> [w224]
            tunnel: w197 -> [w223]
            tunnel: w195 -> [w221]
            tunnel: w192 -> [w220]
            tunnel: w194 -> [w219]
            tunnel: w193 -> [w218]
            tunnel: w203 -> [w217]
            tunnel: [w216] -> w202
            tunnel: w199 -> [w233]
            tunnel: w200 -> [w232]
            tunnel: w202 -> [w231]
            tunnel: w198 -> [w230]
            tunnel: w197 -> [w229]
            tunnel: [w228] -> w201
            tunnel: w196 -> [w227]
            tunnel: w201 -> [w250]
            tunnel: [w248] -> w184
            tunnel: w200 -> [w247]
            tunnel: w199 -> [w246]
            tunnel: w198 -> [w245]
            tunnel: w197 -> [w244]
            frame #0 {
              n134 = call "ReadTemp.vi"("error in (no error)"=w207, "Port Number"=w210, "IP Address"=w211) -> ("error out"=w208:errorcluster, "Temperature"=w209:dbl)  [unwired: 7 in]
            }
            frame #1 {
              n135 = call "Time Delay10"("error in (no error)"=w213, "Delay Time (s)"=1.0) -> ("error out"=w212:errorcluster)  [unwired: 9 in]
            }
            frame #2 {
              n136 = call "TempRampDoubleHeater.vi"("IP Address Heater 1"=w226, "Port Number Heater 1"=w225, "IP Address Heater 2"=w224, "Port Number Heater 2"=w223, "Start T1 (C)"=w222, "End T1 (C)"=w221, "Duration of Ramp (min)"=w219, "Additional Temperature for Heater 2"=w220, "Temperature Log Interval (s)"=w218, "Error In (no error)"=w217) -> ("Error Out"=w216:errorcluster)  [unwired: 3 in, 6 out]
            }
            frame #3 {
              n137 = case shown="False" w227 {
                tunnel: w233 -> [_ w243]
                tunnel: w232 -> [_ w242]
                tunnel: w231 -> [w234 w237]
                tunnel: w230 -> [_ w241]
                tunnel: w229 -> [_ w240]
                tunnel: [w234 w235] -> w228
                frame False {
                }
                frame True {
                  n138 = call "WriteSetPoint.vi"("error in (no error)"=w237, "Setpoint (C)"=25.0, "Port Number"=w243, "IP Address"=w242) -> ("error out"=w236:errorcluster)  [unwired: 6 in, 1 out]
                  n139 = call "WriteSetPoint.vi"("error in (no error)"=w236, "Setpoint (C)"=30.0, "Port Number"=w240, "IP Address"=w241) -> ("error out"=w235:errorcluster)  [unwired: 6 in, 1 out]
                }
              }
            }
            frame #4 {
              n140 = call "EnableStandby.vi"("error in (no error)"=w250, "Port Number"=w246, "IP Address"=w247) -> ("error out"=w249:errorcluster)  [unwired: 7 in, 1 out]
              n141 = call "EnableStandby.vi"("error in (no error)"=w249, "Port Number"=w244, "IP Address"=w245) -> ("error out"=w248:errorcluster)  [unwired: 7 in, 1 out]
            }
          }
          n142 = local read "Ramp Down Duration (min)"() -> (w194:dbl)
          n143 = local read "Final Cold Heater 1 Temperature (C)"() -> (w195:dbl)
          n144 = local read "Additional Temp for Heater 2"() -> (w192:dbl)
          n145 = local read "Set To Room Temp?"() -> (w196:bool)
        }
        frame #1 {
          w251 = FALSE ("Visible")
          # "Waiting for the timer to click"
          n146 = local write "Oven Ramp Down Status (ON/OFF)"(FALSE ("Oven Ramp Down Status (ON/OFF)")) -> ()
          n147 = local read "Next Weekday"() -> (w270:bool)
          n148 = Get Date/Time In Seconds() -> (seconds since 1Jan1904=w282:timestamp)
          n149 = Seconds To Date/Time(time stamp (now)=w282) -> (date time rec=w284:T1)  [unwired: 1 in]
          n150 = local read "Turn ON Minute"() -> (w259:i32)
          n151 = local read "Turn ON Hour"() -> (w260:i32)
          n152 = Unbundle By Name(w284) -> ("fractional second"=w289:dbl, "second"=w288:i32, "day of month"=w281:i32, "month"=w279:i32, "year"=w277:i32, "day of week"=w287:i32, "day of year"=w286:i32, "DST"=w285:i32)  [unwired: 2 out]
          n153 = case shown="True" w270 {
            tunnel: w282 -> [_ w310]
            tunnel: w281 -> [_ w299]
            tunnel: [w292 w297] -> w280
            tunnel: w279 -> [_ w296]
            tunnel: [w291 w296] -> w278
            tunnel: w277 -> [_ w295]
            tunnel: [w290 w295] -> w276
            tunnel: w258 -> [w293 w294]
            tunnel: [w293 w294] -> w271
            frame False {
              n154 = local read "Month"() -> (w291:i32)
              n155 = local read "Day"() -> (w292:i32)
              n156 = local read "Year"() -> (w290:i32)
            }
            frame True {
              n157 = Format Date/Time String(time format string (%c)="%A", seconds (now)=w310) -> (date/time string=w307:string)  [unwired: 1 in]
              n158 = Equal?(x=w307, y="Saturday") -> (x = y?=w303:bool)
              n159 = Select(t=2, s=w303, f=1) -> (s? t:f=w300:i32)
              n160 = Equal?(x=w307, y="Friday") -> (x = y?=w305:bool)
              n161 = Select(t=3, s=w305, f=w300) -> (s? t:f=w298:i32)
              n162 = Add(x=w299, y=w298) -> (x+y=w297:i32)
            }
          }
          n163 = Bundle By Name(cluster=w284, "fractional second"=w289, "second"=w288, "minute"=w259, "hour"=w260, "day of month"=w280, "month"=w278, "year"=w276, "day of week"=w287, "day of year"=w286, "DST"=w285) -> (w283:T1)
          n164 = Date/Time To Seconds(2:w283) -> (0:w274:timestamp)  [unwired: 1 in]
          n165 = Get Date/Time String(date format (0)=enum16{"short", "long", "abbreviated"}."long", seconds (now)=w274, want seconds? (F)=FALSE) -> (date string=w269:string, time string=w268:string)
          n166 = local read "IP Address Heater 1"() -> (w264:string)
          n167 = local read "Port Number Heater 1"() -> (w263:u16)
          n168 = local write "Oven Ramp ON Date"(w269) -> ()
          n169 = local write "Oven Ramp ON Time"(w268) -> ()
          n170 = local read "Temperature Log Interval (s)"() -> (w266:dbl)
          n171 = local read "IP Address Heater 2"() -> (w261:string)
          n172 = local read "Port Number Heater 2"() -> (w262:u16)
          n173 = Multiply(x=w266, y=1000.0) -> (x*y=w265:dbl)
          n174 = while {
            tunnel: w274 -> [w346]
            tunnel: [w325] -> w275
            shift-right: [w311] -> w252
            shift-left: w271 -> [w321]
            tunnel: w265 -> [w324]
            tunnel: w264 -> [w318]
            tunnel: w263 -> [w317]
            tunnel: w262 -> [w316]
            tunnel: w261 -> [w315]
            stop <- w325 stop-if-true
            w322 = u16 1 items=["Sodium Cup (T1)", "Flange (T2)"] ("Thermocouple")
            w323 = u16 0 items=["Sodium Cup (T1)", "Flange (T2)"] ("Thermocouple")
            n175 = Get Date/Time In Seconds() -> (seconds since 1Jan1904=w347:timestamp)
            n176 = Seconds To Date/Time(time stamp (now)=w346) -> (date time rec=w345:T1)  [unwired: 1 in]
            n177 = Seconds To Date/Time(time stamp (now)=w347) -> (date time rec=w344:T1)  [unwired: 1 in]
            n178 = Unbundle By Name(w345) -> ("year"=w342:i32, "month"=w340:i32, "day of month"=w338:i32, "hour"=w336:i32, "minute"=w334:i32)
            n179 = Unbundle By Name(w344) -> ("year"=w343:i32, "month"=w341:i32, "day of month"=w339:i32, "hour"=w337:i32, "minute"=w335:i32)
            n180 = call "ReadTemp.vi"("error in (no error)"=w321, "Port Number"=w317, "IP Address"=w318) -> ("error out"=w312:errorcluster, "Temperature"=w320:dbl)  [unwired: 7 in]
            n181 = local write "T1 (C)"(w320) -> ()
            n182 = Equal?(x=w343, y=w342) -> (x = y?=w333:bool)
            n183 = call "NaOvenTempToInflux.vi"("error in (no error)"=w312, "Temperature Input"=w320, "Thermocouple"=w323) -> ("InfluxDB Comm Error"=w314:bool)  [unwired: 1 in, 1 out]
            n184 = Equal?(x=w341, y=w340) -> (x = y?=w332:bool)
            n185 = Equal?(x=w337, y=w336) -> (x = y?=w331:bool)
            n186 = Equal?(x=w339, y=w338) -> (x = y?=w328:bool)
            n187 = And(x=w333, y=w332) -> (x .and. y?=w329:bool)
            n188 = call "ReadTemp.vi"("error in (no error)"=w312, "Port Number"=w316, "IP Address"=w315) -> ("error out"=w311:errorcluster, "Temperature"=w319:dbl)  [unwired: 7 in]
            n189 = And(x=w329, y=w328) -> (x .and. y?=w327:bool)
            n190 = Equal?(x=w335, y=w334) -> (x = y?=w330:bool)
            n191 = local write "T2 (C)"(w319) -> ()
            n192 = And(x=w331, y=w330) -> (x .and. y?=w326:bool)
            n193 = local write "Update to Influx (T1)"(w314) -> ()
            n194 = call "NaOvenTempToInflux.vi"("error in (no error)"=w311, "Temperature Input"=w319, "Thermocouple"=w322) -> ("InfluxDB Comm Error"=w313:bool)  [unwired: 1 in, 1 out]
            n195 = And(x=w327, y=w326) -> (x .and. y?=w325:bool)
            n196 = local write "Update to Influx (T2)"(w313) -> ()
            n197 = Wait (ms)(milliseconds to wait=w324) -> ()  [unwired: 1 out]
          }
          n198 = property on="Update to Influx (T2)" class="Bool (strict)"(error in=w252, "Visible"=w251) -> (error out=w253:errorcluster)  [unwired: 1 in, 1 out]
          n199 = property on="Update to Influx (T1)" class="Bool (strict)"(error in=w253, "Visible"=w251) -> (error out=w254:errorcluster)  [unwired: 1 in, 1 out]
          n200 = property on="T1 (C)" class="DigNum (strict)"(error in=w254, "Visible"=w251) -> (error out=w255:errorcluster)  [unwired: 1 in, 1 out]
          n201 = property on="T2 (C)" class="DigNum (strict)"(error in=w255, "Visible"=w251) -> (error out=w256:errorcluster)  [unwired: 1 in, 1 out]
          n202 = local write "Oven Ramp Up Status (ON/OFF)"(w275) -> ()
        }
        frame #2 {
          # "5. Perform Ramp"
          # "3. Setting up the device to perform the ramp"
          # "2. Choosing the right start temperature"
          n203 = local read "Port Number Heater 1"() -> (w359:u16)
          n204 = local read "IP Address Heater 1"() -> (w360:string)
          n205 = local read "Port Number Heater 2"() -> (w357:u16)
          n206 = local read "Additional Temp for Heater 2"() -> (w356:dbl)
          n207 = local read "IP Address Heater 2"() -> (w358:string)
          n208 = call "Time Delay"("error in (no error)"=w350, "Delay Time (s)"=1.0) -> ("error out"=w349:errorcluster)  [unwired: 9 in]
          n209 = call "DisableStandby.vi"("error in (no error)"=w349, "Port Number"=w359, "IP Address"=w360) -> ("error out"=w362:errorcluster)  [unwired: 7 in, 1 out]
          n210 = call "DisableStandby.vi"("error in (no error)"=w362, "Port Number"=w357, "IP Address"=w358) -> ("error out"=w361:errorcluster)  [unwired: 7 in, 1 out]
          n211 = call "ReadTemp.vi"("error in (no error)"=w361, "Port Number"=w359, "IP Address"=w360) -> ("error out"=w375:errorcluster, "Temperature"=w372:dbl)  [unwired: 7 in]
          n212 = call "ReadTemp.vi"("error in (no error)"=w375, "Port Number"=w357, "IP Address"=w358) -> ("error out"=w370:errorcluster, "Temperature"=w374:dbl)  [unwired: 7 in]
          n213 = Subtract(x=w374, y=w356) -> (x-y=w371:dbl)
          n214 = Greater?(x=w372, y=w371) -> (0:w373:bool)
          n215 = Select(t=w372, s=w373, f=w371) -> (s? t:f=w369:dbl)
          n216 = Add(x=2.0, y=w369) -> (x+y=w367:dbl)
          n217 = call "WriteSetPoint.vi"("error in (no error)"=w370, "Setpoint (C)"=w367, "Port Number"=w359, "IP Address"=w360) -> ("error out"=w380:errorcluster)  [unwired: 6 in, 1 out]
          n218 = Add(x=w367, y=w356) -> (x+y=w381:dbl)
          n219 = call "WriteSetPoint.vi"("error in (no error)"=w380, "Setpoint (C)"=w381, "Port Number"=w357, "IP Address"=w358) -> ("error out"=w379:errorcluster)  [unwired: 6 in, 1 out]
          n220 = call "WriteConfgInpt_KtypeTC.vi"("error in (no error)"=w379, "Port Number"=w359, "IP Address"=w360) -> ("error out"=w378:errorcluster)  [unwired: 7 in, 1 out]
          n221 = call "WriteConfgInpt_KtypeTC.vi"("error in (no error)"=w378, "Port Number"=w357, "IP Address"=w358) -> ("error out"=w377:errorcluster)  [unwired: 7 in, 1 out]
          n222 = call "WriteConfgRDG_Dec1Celcius.vi"("error in (no error)"=w377, "Port Number"=w359, "IP Address"=w360) -> ("error out"=w376:errorcluster)  [unwired: 7 in, 1 out]
          n223 = call "WriteConfgRDG_Dec1Celcius.vi"("error in (no error)"=w376, "Port Number"=w357, "IP Address"=w358) -> ("error out"=w348:errorcluster)  [unwired: 7 in, 1 out]
          n224 = call "Reset.vi"("error in (no error)"=w348, "Port Number"=w359, "IP Address"=w360) -> ("error out"=w366:errorcluster)  [unwired: 7 in, 1 out]
          n225 = call "Reset.vi"("error in (no error)"=w366, "Port Number"=w357, "IP Address"=w358) -> ("error out"=w365:errorcluster)  [unwired: 7 in, 1 out]
          n226 = local read "Final Hot Heater 1 Temperature (C)"() -> (w353:dbl)
          n227 = local read "Temperature Log Interval (s)"() -> (w354:dbl)
          n228 = local read "Ramp Up Duration (min)"() -> (w355:dbl)
          n229 = call "Time Delay9"("error in (no error)"=w365, "Delay Time (s)"=5.0) -> ("error out"=w364:errorcluster)  [unwired: 9 in]
          n230 = call "TempRampDoubleHeater.vi"("IP Address Heater 1"=w360, "Port Number Heater 1"=w359, "IP Address Heater 2"=w358, "Port Number Heater 2"=w357, "Start T1 (C)"=w367, "End T1 (C)"=w353, "Duration of Ramp (min)"=w355, "Additional Temperature for Heater 2"=w356, "Temperature Log Interval (s)"=w354, "Error In (no error)"=w364) -> ("Error Out"=w352:errorcluster)  [unwired: 3 in, 6 out]
        }
        frame #3 {
          w382 = TRUE ("Visible")
          n231 = property on="Update to Influx (T2)" class="Bool (strict)"(error in=w387, "Visible"=w382) -> (error out=w386:errorcluster)  [unwired: 1 in, 1 out]
          n232 = property on="Update to Influx (T1)" class="Bool (strict)"(error in=w386, "Visible"=w382) -> (error out=w385:errorcluster)  [unwired: 1 in, 1 out]
          n233 = local write "Oven Ramp Up Status (ON/OFF)"(FALSE ("Oven Ramp Up Status (ON/OFF)")) -> ()
          n234 = property on="T1 (C)" class="DigNum (strict)"(error in=w385, "Visible"=w382) -> (error out=w384:errorcluster)  [unwired: 1 in, 1 out]
          n235 = local read "Temperature Log Interval (s)"() -> (w394:dbl)
          n236 = property on="T2 (C)" class="DigNum (strict)"(error in=w384, "Visible"=w382) -> (error out=w383:errorcluster)  [unwired: 1 in, 1 out]
          n237 = local read "IP Address Heater 1"() -> (w393:string)
          n238 = local read "Port Number Heater 1"() -> (w392:u16)
          n239 = local read "IP Address Heater 2"() -> (w391:string)
          n240 = local read "Port Number Heater 2"() -> (w390:u16)
          n241 = while {
            tunnel: w394 -> [w408]
            tunnel: w393 -> [w410]
            tunnel: w392 -> [w409]
            shift-right: [w395] -> w389
            shift-left: w383 -> [w406]
            tunnel: w391 -> [w404]
            tunnel: w390 -> [w403]
            stop <- FALSE stop-if-true
            w401 = u16 1 items=["Sodium Cup (T1)", "Flange (T2)"] ("Thermocouple")
            w402 = u16 0 items=["Sodium Cup (T1)", "Flange (T2)"] ("Thermocouple")
            n242 = Multiply(x=1000.0 ("y"), y=w408) -> (x*y=w411:dbl)
            n243 = call "ReadTemp.vi"("error in (no error)"=w406, "Port Number"=w409, "IP Address"=w410) -> ("error out"=w396:errorcluster, "Temperature"=w400:dbl)  [unwired: 7 in]
            n244 = Wait (ms)(milliseconds to wait=w411) -> ()  [unwired: 1 out]
            n245 = local write "T1 (C)"(w400) -> ()
            n246 = call "NaOvenTempToInflux.vi"("error in (no error)"=w396, "Temperature Input"=w400, "Thermocouple"=w402) -> ("InfluxDB Comm Error"=w398:bool)  [unwired: 1 in, 1 out]
            n247 = local write "Update to Influx (T1)"(w398) -> ()
            n248 = call "ReadTemp.vi"("error in (no error)"=w396, "Port Number"=w403, "IP Address"=w404) -> ("error out"=w395:errorcluster, "Temperature"=w399:dbl)  [unwired: 7 in]
            n249 = local write "T2 (C)"(w399) -> ()
            n250 = call "NaOvenTempToInflux.vi"("error in (no error)"=w395, "Temperature Input"=w399, "Thermocouple"=w401) -> ("InfluxDB Comm Error"=w397:bool)  [unwired: 1 in, 1 out]
            n251 = local write "Update to Influx (T2)"(w397) -> ()
          }
        }
      }
    }
    frame 2 {
      n252 = stacked-sequence {
        seq-local: [w424 _] -> [_ w489]
        tunnel: w413 -> [w421 _]
        tunnel: [_ w491] -> w412
        frame #0 {
          w417 = FALSE ("Visible")
          n253 = property on="Update to Influx (T2)" class="Bool (strict)"(error in=w421, "Visible"=w417) -> (error out=w420:errorcluster)  [unwired: 1 in, 1 out]
          n254 = property on="Update to Influx (T1)" class="Bool (strict)"(error in=w420, "Visible"=w417) -> (error out=w419:errorcluster)  [unwired: 1 in, 1 out]
          n255 = property on="T1 (C)" class="DigNum (strict)"(error in=w419, "Visible"=w417) -> (error out=w418:errorcluster)  [unwired: 1 in, 1 out]
          n256 = property on="T2 (C)" class="DigNum (strict)"(error in=w418, "Visible"=w417) -> (error out=w416:errorcluster)  [unwired: 1 in, 1 out]
          n257 = property on="Oven Ramp ON Date" class="Str"(error in=w416, "Visible"=w417) -> (error out=w415:errorcluster)  [unwired: 1 in, 1 out]
          n258 = local write "Oven Ramp Up Status (ON/OFF)"(FALSE ("Oven Ramp Up Status (ON/OFF)")) -> ()
          n259 = local write "Oven Ramp Down Status (ON/OFF)"(TRUE ("Oven Ramp Down Status (ON/OFF)")) -> ()
          n260 = property on="Oven Ramp ON Time" class="Str"(error in=w415, "Visible"=w417) -> (error out=w414:errorcluster)  [unwired: 1 in, 1 out]
          n261 = local read "IP Address Heater 2"() -> (w431:string)
          n262 = local read "Port Number Heater 2"() -> (w430:u16)
          n263 = local read "Port Number Heater 1"() -> (w432:u16)
          n264 = local read "IP Address Heater 1"() -> (w433:string)
          n265 = local read "Temperature Log Interval (s)"() -> (w426:dbl)
          n266 = flat-sequence {
            tunnel: w433 -> [w444]
            tunnel: w432 -> [w443]
            tunnel: w414 -> [w440]
            tunnel: [w442] -> w439
            tunnel: [w441] -> w438
            tunnel: w439 -> [w448]
            tunnel: w438 -> [w446]
            tunnel: [w448] -> w437
            tunnel: [w445] -> w436
            tunnel: w437 -> [w455]
            tunnel: w433 -> [w459]
            tunnel: w432 -> [w458]
            tunnel: w431 -> [w457]
            tunnel: w430 -> [w456]
            tunnel: w428 -> [w454]
            tunnel: w425 -> [w453]
            tunnel: w427 -> [w452]
            tunnel: w426 -> [w451]
            tunnel: w436 -> [w450]
            tunnel: [w449] -> w435
            tunnel: w432 -> [w466]
            tunnel: w433 -> [w465]
            tunnel: w435 -> [w464]
            tunnel: w431 -> [w463]
            tunnel: w430 -> [w462]
            tunnel: [w461] -> w434
            tunnel: w429 -> [w460]
            tunnel: w434 -> [w483]
            tunnel: [w481] -> w424
            tunnel: w433 -> [w480]
            tunnel: w432 -> [w479]
            tunnel: w431 -> [w478]
            tunnel: w430 -> [w477]
            frame #0 {
              n267 = call "ReadTemp.vi"("error in (no error)"=w440, "Port Number"=w443, "IP Address"=w444) -> ("error out"=w441:errorcluster, "Temperature"=w442:dbl)  [unwired: 7 in]
            }
            frame #1 {
              n268 = call "Time Delay11"("error in (no error)"=w446, "Delay Time (s)"=1.0) -> ("error out"=w445:errorcluster)  [unwired: 9 in]
            }
            frame #2 {
              n269 = call "TempRampDoubleHeater.vi"("IP Address Heater 1"=w459, "Port Number Heater 1"=w458, "IP Address Heater 2"=w457, "Port Number Heater 2"=w456, "Start T1 (C)"=w455, "End T1 (C)"=w454, "Duration of Ramp (min)"=w452, "Additional Temperature for Heater 2"=w453, "Temperature Log Interval (s)"=w451, "Error In (no error)"=w450) -> ("Error Out"=w449:errorcluster)  [unwired: 3 in, 6 out]
            }
            frame #3 {
              n270 = case shown="False" w460 {
                tunnel: w466 -> [_ w476]
                tunnel: w465 -> [_ w475]
                tunnel: w464 -> [w467 w470]
                tunnel: w463 -> [_ w474]
                tunnel: w462 -> [_ w473]
                tunnel: [w467 w468] -> w461
                frame False {
                }
                frame True {
                  n271 = call "WriteSetPoint.vi"("error in (no error)"=w470, "Setpoint (C)"=25.0, "Port Number"=w476, "IP Address"=w475) -> ("error out"=w469:errorcluster)  [unwired: 6 in, 1 out]
                  n272 = call "WriteSetPoint.vi"("error in (no error)"=w469, "Setpoint (C)"=30.0, "Port Number"=w473, "IP Address"=w474) -> ("error out"=w468:errorcluster)  [unwired: 6 in, 1 out]
                }
              }
            }
            frame #4 {
              n273 = call "EnableStandby.vi"("error in (no error)"=w483, "Port Number"=w479, "IP Address"=w480) -> ("error out"=w482:errorcluster)  [unwired: 7 in, 1 out]
              n274 = call "EnableStandby.vi"("error in (no error)"=w482, "Port Number"=w477, "IP Address"=w478) -> ("error out"=w481:errorcluster)  [unwired: 7 in, 1 out]
            }
          }
          n275 = local read "Ramp Down Duration (min)"() -> (w427:dbl)
          n276 = local read "Final Cold Heater 1 Temperature (C)"() -> (w428:dbl)
          n277 = local read "Additional Temp for Heater 2"() -> (w425:dbl)
          n278 = local read "Set To Room Temp?"() -> (w429:bool)
        }
        frame #1 {
          w484 = TRUE ("Visible")
          n279 = property on="Update to Influx (T2)" class="Bool (strict)"(error in=w489, "Visible"=w484) -> (error out=w488:errorcluster)  [unwired: 1 in, 1 out]
          n280 = property on="Update to Influx (T1)" class="Bool (strict)"(error in=w488, "Visible"=w484) -> (error out=w487:errorcluster)  [unwired: 1 in, 1 out]
          n281 = property on="T1 (C)" class="DigNum (strict)"(error in=w487, "Visible"=w484) -> (error out=w486:errorcluster)  [unwired: 1 in, 1 out]
          n282 = property on="T2 (C)" class="DigNum (strict)"(error in=w486, "Visible"=w484) -> (error out=w485:errorcluster)  [unwired: 1 in, 1 out]
          n283 = local write "Oven Ramp Down Status (ON/OFF)"(FALSE ("Oven Ramp Up Status (ON/OFF)")) -> ()
          n284 = local read "Temperature Log Interval (s)"() -> (w496:dbl)
          n285 = local read "IP Address Heater 1"() -> (w495:string)
          n286 = local read "Port Number Heater 1"() -> (w494:u16)
          n287 = local read "IP Address Heater 2"() -> (w493:string)
          n288 = local read "Port Number Heater 2"() -> (w492:u16)
          n289 = while {
            tunnel: w496 -> [w510]
            tunnel: w495 -> [w512]
            tunnel: w494 -> [w511]
            shift-right: [w497] -> w491
            shift-left: w485 -> [w508]
            tunnel: w493 -> [w506]
            tunnel: w492 -> [w505]
            stop <- FALSE stop-if-true
            w503 = u16 1 items=["Sodium Cup (T1)", "Flange (T2)"] ("Thermocouple")
            w504 = u16 0 items=["Sodium Cup (T1)", "Flange (T2)"] ("Thermocouple")
            n290 = Multiply(x=1000.0 ("y"), y=w510) -> (x*y=w513:dbl)
            n291 = call "ReadTemp.vi"("error in (no error)"=w508, "Port Number"=w511, "IP Address"=w512) -> ("error out"=w498:errorcluster, "Temperature"=w502:dbl)  [unwired: 7 in]
            n292 = Wait (ms)(milliseconds to wait=w513) -> ()  [unwired: 1 out]
            n293 = local write "T1 (C)"(w502) -> ()
            n294 = call "NaOvenTempToInflux.vi"("error in (no error)"=w498, "Temperature Input"=w502, "Thermocouple"=w504) -> ("InfluxDB Comm Error"=w500:bool)  [unwired: 1 in, 1 out]
            n295 = local write "Update to Influx (T1)"(w500) -> ()
            n296 = call "ReadTemp.vi"("error in (no error)"=w498, "Port Number"=w505, "IP Address"=w506) -> ("error out"=w497:errorcluster, "Temperature"=w501:dbl)  [unwired: 7 in]
            n297 = local write "T2 (C)"(w501) -> ()
            n298 = call "NaOvenTempToInflux.vi"("error in (no error)"=w497, "Temperature Input"=w501, "Thermocouple"=w503) -> ("InfluxDB Comm Error"=w499:bool)  [unwired: 1 in, 1 out]
            n299 = local write "Update to Influx (T2)"(w499) -> ()
          }
        }
      }
    }
    frame 0, Default {
      w514 = FALSE ("Visible")
      w518 = TRUE ("Visible")
      n300 = property on="Update to Influx (T1)" class="Bool (strict)"(error in=w522, "Visible"=w518) -> (error out=w521:errorcluster)  [unwired: 1 in, 1 out]
      n301 = property on="Update to Influx (T2)" class="Bool (strict)"(error in=w521, "Visible"=w518) -> (error out=w520:errorcluster)  [unwired: 1 in, 1 out]
      n302 = local write "Oven Ramp Up Status (ON/OFF)"(FALSE ("Oven Ramp Up Status (ON/OFF)")) -> ()
      n303 = local write "Oven Ramp Down Status (ON/OFF)"(FALSE ("Oven Ramp Down Status (ON/OFF)")) -> ()
      n304 = property on="T1 (C)" class="DigNum (strict)"(error in=w520, "Visible"=w518) -> (error out=w519:errorcluster)  [unwired: 1 in, 1 out]
      n305 = property on="T2 (C)" class="DigNum (strict)"(error in=w519, "Visible"=w518) -> (error out=w517:errorcluster)  [unwired: 1 in, 1 out]
      n306 = property on="Oven Ramp ON Date" class="Str"(error in=w517, "Visible"=w514) -> (error out=w516:errorcluster)  [unwired: 1 in, 1 out]
      n307 = property on="Oven Ramp ON Time" class="Str"(error in=w516, "Visible"=w514) -> (error out=w515:errorcluster)  [unwired: 1 in, 1 out]
      n308 = local read "Temperature Log Interval (s)"() -> (w529:dbl)
      n309 = local read "IP Address Heater 1"() -> (w528:string)
      n310 = local read "Port Number Heater 1"() -> (w527:u16)
      n311 = local read "IP Address Heater 2"() -> (w526:string)
      n312 = local read "Port Number Heater 2"() -> (w525:u16)
      n313 = while {
        tunnel: w529 -> [w544]
        tunnel: w528 -> [w546]
        tunnel: w527 -> [w545]
        shift-right: [w531] -> w530
        shift-left: w515 -> [w542]
        tunnel: w526 -> [w540]
        tunnel: w525 -> [w539]
        stop <- FALSE stop-if-true
        w537 = u16 1 items=["Sodium Cup (T1)", "Flange (T2)"] ("Thermocouple")
        w538 = u16 0 items=["Sodium Cup (T1)", "Flange (T2)"] ("Thermocouple")
        n314 = Multiply(x=1000.0 ("y"), y=w544) -> (x*y=w547:dbl)
        n315 = call "ReadTemp.vi"("error in (no error)"=w542, "Port Number"=w545, "IP Address"=w546) -> ("error out"=w532:errorcluster, "Temperature"=w536:dbl)  [unwired: 7 in]
        n316 = Wait (ms)(milliseconds to wait=w547) -> ()  [unwired: 1 out]
        n317 = local write "T1 (C)"(w536) -> ()
        n318 = call "NaOvenTempToInflux.vi"("error in (no error)"=w532, "Temperature Input"=w536, "Thermocouple"=w538) -> ("InfluxDB Comm Error"=w534:bool)  [unwired: 1 in, 1 out]
        n319 = local write "Update to Influx (T1)"(w534) -> ()
        n320 = call "ReadTemp.vi"("error in (no error)"=w532, "Port Number"=w539, "IP Address"=w540) -> ("error out"=w531:errorcluster, "Temperature"=w535:dbl)  [unwired: 7 in]
        n321 = local write "T2 (C)"(w535) -> ()
        n322 = call "NaOvenTempToInflux.vi"("error in (no error)"=w531, "Temperature Input"=w535, "Thermocouple"=w537) -> ("InfluxDB Comm Error"=w533:bool)  [unwired: 1 in, 1 out]
        n323 = local write "Update to Influx (T2)"(w533) -> ()
      }
    }
  }
  "Error Out" <- w3
